vi "Statistical Metrics.vi"(1 "ET Array":dbl[](array[numeric]), 3 "base path":path) -> (7 "Histogram Graph":T1, 8 "Statistical Metrics":T2, 10 "Error Out":errorcluster)   [LabVIEW 2020]
uses:
  <vilib>/Analysis/NI_AALBase.lvlib
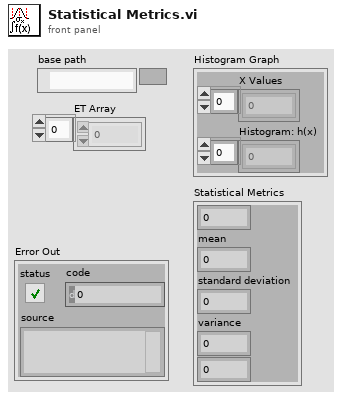
[diagram p1: front panel]
types:
  T1 = cluster{"X Values":dbl[], "Histogram: h(x)":i32[]}
  T2 = cluster{dbl, "mean":dbl, "standard deviation":dbl, "variance":dbl, dbl}
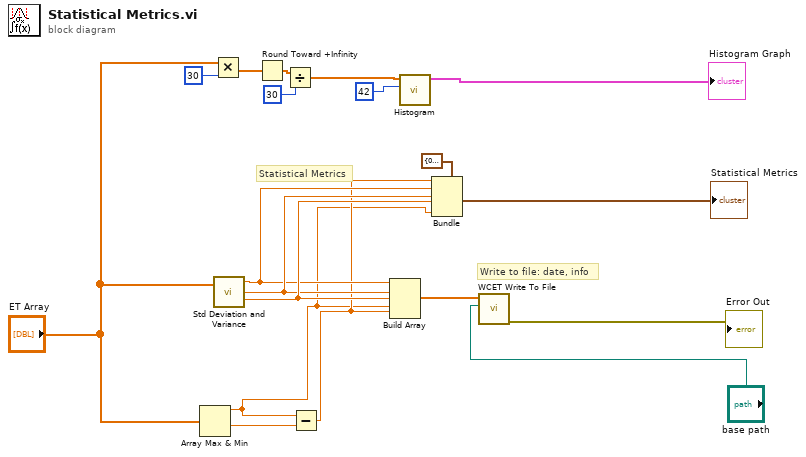
[diagram p0: block diagram]
diagram:
  # "Write to file: date, info"
  # "Statistical Metrics"
  n1 = Array Max & Min(array="ET Array") -> (max value=w12:dbl, min value=w1:dbl)  [unwired: 2 out]
  n2 = Multiply(x="ET Array", y=30) -> (x*y=w7:dbl[])
  n3 = call <vilib>:"Std Deviation and Variance.vi"("X"="ET Array") -> ("mean"=w14:dbl, "standard deviation"=w15:dbl, "variance"=w16:dbl)  [unwired: 1 in]
  n4 = Round Toward +Infinity(x=w7) -> (ceil(x): smallest int >= x=w8:dbl[])
  n5 = Divide(x=w8, y=30) -> (x/y=w10:dbl[])
  n6 = Subtract(x=w12, y=w1) -> (x-y=w13:dbl)
  n7 = Build Array(w14, w15, w16, w12, w13) -> (w2:dbl[])
  n8 = call <vilib>:"Histogram.vi"("intervals"=42, "X"=w10) -> ("Histogram Graph"=→"Histogram Graph":T1)  [unwired: 6 in, 3 out]
  n9 = Bundle(cluster=T2 {0.0, "mean"=0.0, "standard deviation"=0.0, "variance"=0.0, 0.0}, w13, "mean"=w14, "standard deviation"=w15, "variance"=w16, w12) -> (→"Statistical Metrics":T2)
  n10 = call "WCET Write To File.vi"("Path"="base path", "Statistical Metrics"=w2) -> ("Error out"=→"Error Out":errorcluster)  [unwired: 9 in]
